vi "Get Session Info - 1Sess .vi"(8 "error in":errorcluster, 11 "session reservation in":refnum<class "Session Reservation.lvclass">) -> (0 "error out":errorcluster, 2 "session info":T1, 3 "session reservation out":refnum<class "Session Reservation.lvclass">)   [LabVIEW 2020, in "MeasurementLink Session Management.lvlib" / "Session Reservation.lvclass"]
doc: "Gets the connection information for the given <b>pin type</b>, <b>pin or relay name</b>, <b>instrument</b>, and <b>site</b>.The <b>instrument</b> input must return a valid instrument_type_id from the <b>Get Instrument Type ID.vi</b> override. The <b>connection type</b> input should be a cluster with two elements. The first element is a <b>Connection.ctl</b> cluster. The second element is the type of the session."
uses:
  Session Reservation.lvclass
  MeasurementLink Session Management Client/RPC Messages/ni_measurementlink_sessionmanagement_v1_SessionInformation.ctl
  MeasurementLink Session Management Client/RPC Messages/nidevice_grpc_Session.ctl
  MeasurementLink Session Management Client/RPC Messages/ni_measurementlink_sessionmanagement_v1_ChannelMapping.ctl
  Session Reservation.lvclass/Session Reservation.ctl
  Is DVR Valid.vi
  MeasurementLink Measurement Server/Helpers/Error Strings Global Internal.vi
  MeasurementLink Session Management Client/MeasurementLink Session Management Client.lvlib
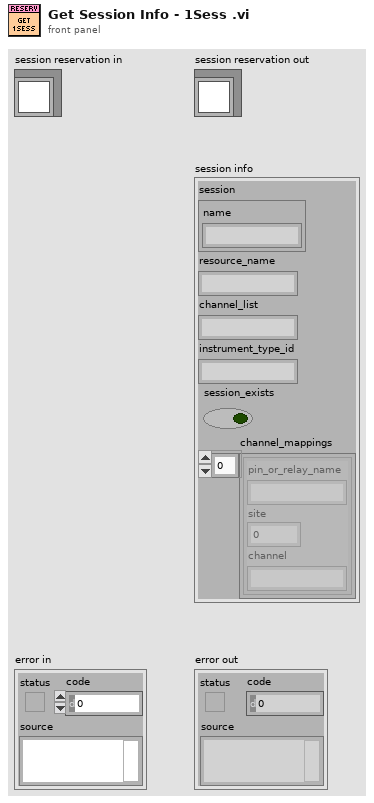
[diagram p1: front panel]
types:
  T1 = typedef "MeasurementLink Session Management Client.lvlib/ni_measurementlink_sessionmanagement_v1_SessionInformation.ctl" = cluster{"session":T2, "resource_name":string, "channel_list":string, "instrument_type_id":string, "session_exists":bool, "channel_mappings":T3[]}
  T2 = typedef "MeasurementLink Session Management Client.lvlib/nidevice_grpc_Session.ctl" = cluster{"name":string}
  T3 = typedef "MeasurementLink Session Management Client.lvlib/ni_measurementlink_sessionmanagement_v1_ChannelMapping.ctl" = cluster{"pin_or_relay_name":string, "site":i32, "channel":string}
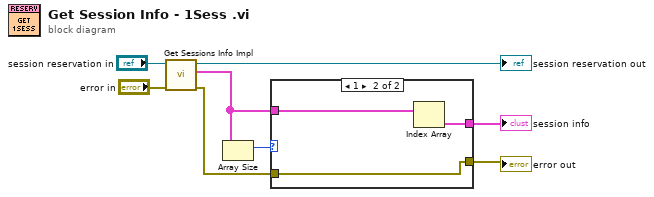
[diagram p0: block diagram]
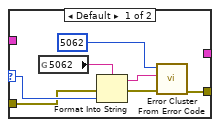
[diagram p2: hidden frame]
diagram:
  n1 = call "Get Sessions Info Impl.vi"("error in"="error in", "session reservation in"="session reservation in") -> ("error out"=w3:errorcluster, "sessions info"=w2:T1[], "session reservation out"=→"session reservation out":refnum<class "Session Reservation.lvclass">)  [unwired: 7 in]
  n2 = Array Size(array=w2) -> (size(s)=w5:i32)
  n3 = case shown="1" w5 {
    selector: w5 -> [w10 _]
    tunnel: w2 -> [_ w18]
    tunnel: [_ w17] -> w1
    tunnel: [w15 w16] -> w4
    tunnel: w3 -> [w9 w16]
    frame Default {
      n4 = global read "Error Strings Global Internal.vi" "5062"() -> (w11:string)
      n5 = Format Into String(format string=w11, error in=w9, w10) -> (resulting string=w12:string, error out=w13:errorcluster)  [unwired: 1 in]
      n6 = call <vilib>:"Error Cluster From Error Code.vi"("error in (no error)"=w13, "error message (\"\")"=w12, "error code (0)"=5062) -> ("error out"=w15:errorcluster)  [unwired: 6 in]
    }
    frame 1 {
      n7 = Index Array(array=w18) -> (element=w17:T1)  [unwired: 1 in]
    }
  }
  "error out" <- w4
  "session info" <- w1
